vi "anti_wind_up_integral_test.vi"() -> ()   [LabVIEW 2014]
uses:
  <vilib>/Platform/TimedLoop/XDataNode/timing_clust.ctl
  <vilib>/Platform/TimedLoop/XDataNode/nitl_modes.ctl
  <vilib>/Platform/TimedLoop/XDataNode/wakeup.ctl
  <vilib>/platform/TimedLoop/XDataNode/XDataNode.xnode
  <vilib>/Platform/TimedLoop/XDataNode/XDNodeRunTimeDep.lvlib
  <vilib>/ptbypt/NI_PtbyPt.lvlib
panel:
  out "Waveform Chart":cluster{"upper limit":dbl, "integral x(t)":dbl}(graph)
  in  "stop":bool
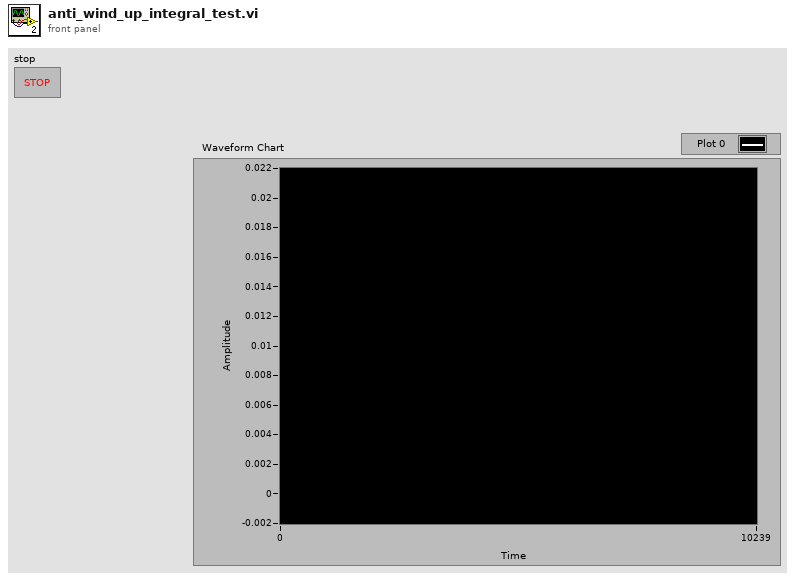
[diagram p1: front panel]
types:
  T1 = typedef "XDNodeRunTimeDep.lvlib/timing_clust.ctl" = cluster{"Expected End [f-1]":u64, "Actual End [f-1]":u64, "Finished Late? [f-1]":bool, "Expected End [i-1]":u64, "Actual End [i-1]":u64, "Finished Late? [i-1]":bool, "Expected Start [i]":u64, "Actual Start [i]":u64, "Expected Start [f]":u64, "Actual Start [f]":u64, "Source Name":string, "Structure Name":string, "Period":i64, "Deadline":i64, "Offset":i64, "Start":i64, "Priority":i32, "Timeout":i32, "Mode":T2, "Wakeup Reason":T3, "Error":errorcluster, "Source Type":string, "Secondary Source Type":string, "Global End Time":u64, "Global Start Time":u64, "Frame Duration":u64, "Iteration Duration":u64, "Assigned CPU":i32, "I/O Scan Engine Mode":u32}
  T2 = typedef "XDNodeRunTimeDep.lvlib/nitl_modes.ctl" = enum32{"No Change", "Process missed periods, maintain original phase", "Discard missed periods, maintain original phase", "Process missed periods, ignore original phase", "Discard missed periods, ignore original phase"}
  T3 = typedef "XDNodeRunTimeDep.lvlib/wakeup.ctl" = enum32{"Normal", "Aborted", "Asynchronous wakeup", "Timing source error", "Timed loop error", "Timeout"}
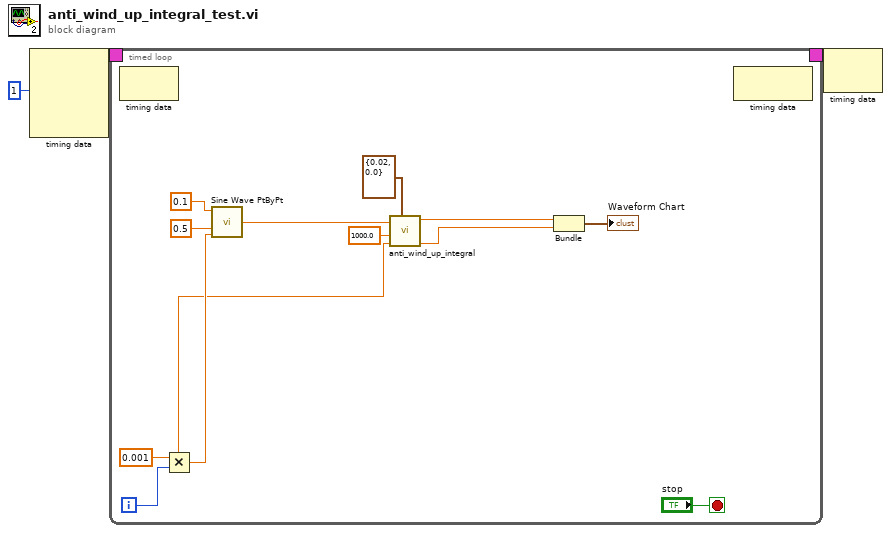
[diagram p0: block diagram]
diagram:
  n1 = node-c288(i64 1 ("Period")) -> (w3:T1)  [unwired: 3 in]
  n2 = timed-loop {
    timing: w3 -> [_]
    timing-out: [_] -> w2
    i -> [w14]
    stop <- "stop" stop-if-true
    w10 = 0.001 ("x")
    n3 = node-c288() -> ()  [unwired: 1 in, 1 out]
    n4 = Multiply(x=w10, y=w14) -> (x*y=w13:dbl)
    n5 = call <vilib>:"Sine Wave PtByPt.vi"("time"=w13, "frequency"=0.5, "amplitude"=0.1) -> ("sine wave"=w5:dbl)  [unwired: 1 in]
    n6 = call "anti_wind_up_integral.vi"("Limits"=cluster{"Upper limit":dbl, "Lower limit ":dbl} {"Upper limit"=0.02, "Lower limit "=0.0}, "Ts"=w10, "Kb"=1000.0, "Input"=w5) -> ("Integral output"=w7:dbl, "Output"=w8:dbl)  [unwired: 6 in]
    n7 = Bundle("Output"=w8, "Integral output"=w7) -> (→"Waveform Chart":cluster{"Output":dbl, "Integral output":dbl})  [unwired: 1 in]
    n8 = node-c288() -> ()  [unwired: 1 in, 1 out]
  }
  n9 = node-c288(w2) -> ()  [unwired: 1 out]
